vi "U3 - Create All Message Queues.vi"(8 "error in (no error)":errorcluster, 11 "Process Name":string="Feed Module 1") -> (0 "error out":errorcluster, 3 "Message Queues out":T1)   [LabVIEW 2018]
uses:
  support/Message Queue/Message Cluster.ctl
  support/Message Queue/Message Queue.lvlib
  support/Message Queue/All Message Queues.ctl
  support/Message Queue/Enqueue Message (Single).vi
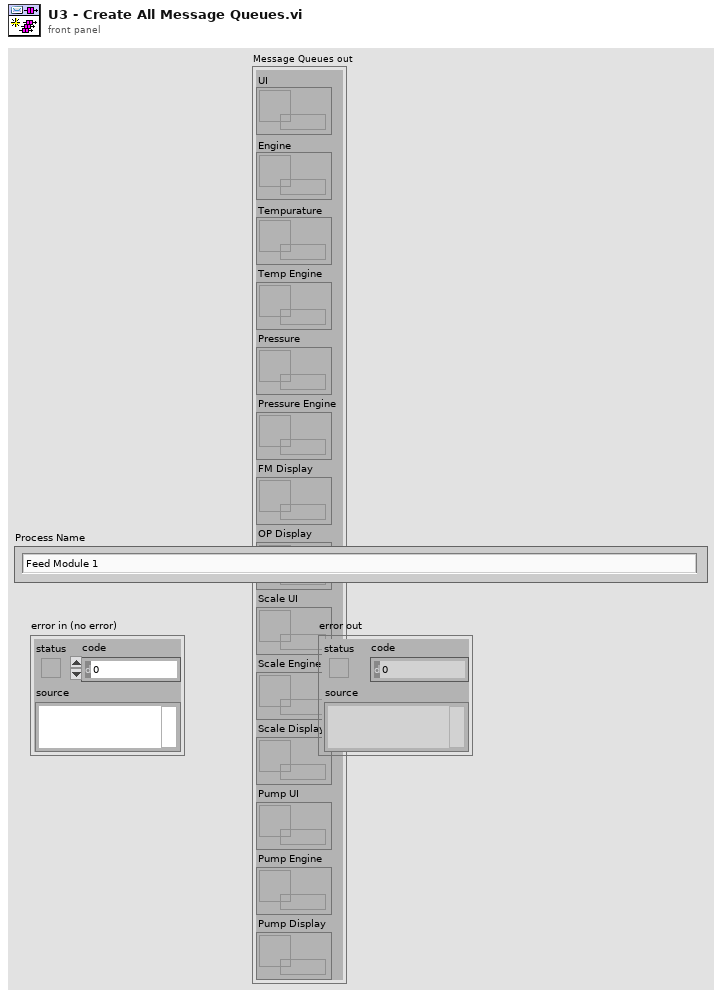
[diagram p1: front panel]
types:
  T1 = typedef "Message Queue.lvlib/All Message Queues.ctl" = cluster{"UI":refnum<queue>, "Engine":refnum<queue>, "Tempurature":refnum<queue>, "Temp Engine":refnum<queue>, "Pressure":refnum<queue>, "Pressure Engine":refnum<queue>, "FM Display":refnum<queue>, "OP Display":refnum<queue>, "Scale UI":refnum<queue>, "Scale Engine":refnum<queue>, "Scale Display":refnum<queue>, "Pump UI":refnum<queue>, "Pump Engine":refnum<queue>, "Pump Display":refnum<queue>}
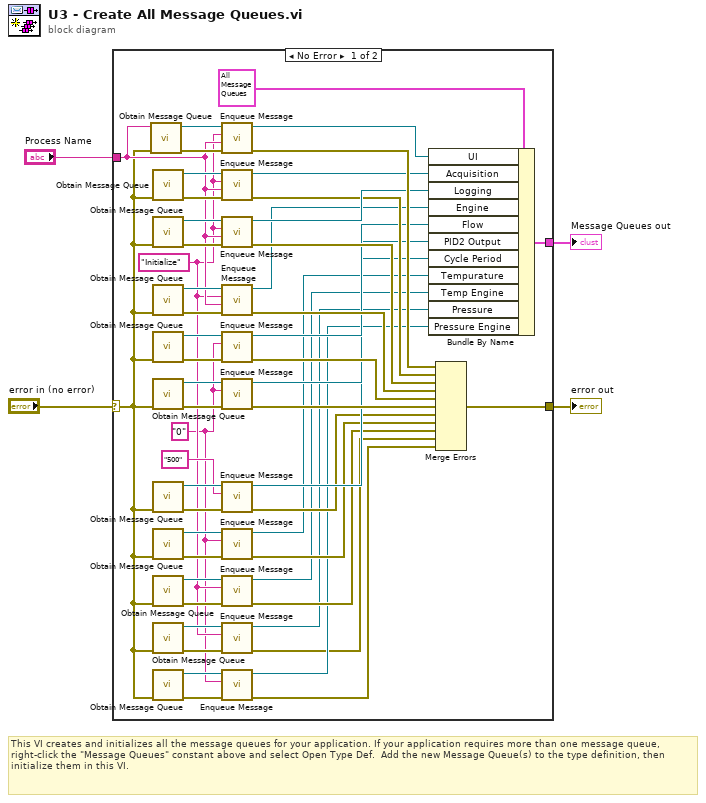
[diagram p0: block diagram]
diagram:
  # "This VI creates and initializes all the message queues for your application. If your application requires more than one message queue, right-click the \"Message Queues\" constant above and select Open Type Def.  Add the new Message Queue(s) to the type definition, then initialize them in this VI."
  n1 = case shown="No Error" "error in (no error)" {
    selector: "error in (no error)" -> [w9 w57]
    tunnel: [w44 w57] -> w4
    tunnel: [w54 _] -> w3
    tunnel: "Process Name" -> [w37 _]
    frame No Error {
      w5 = "0" ("Message")
      w6 = "Initialize" ("Message")
      n2 = call "Obtain Message Queue.vi"("error in (no error)"=w9, "name (unnamed)"=w37) -> ("error out"=w53:errorcluster, "Message Queue"=w52:refnum<queue>)  [unwired: 8 in]
      n3 = call "Obtain Message Queue.vi"("error in (no error)"=w9) -> ("error out"=w50:errorcluster, "Message Queue"=w51:refnum<queue>)  [unwired: 9 in]
      n4 = call "Obtain Message Queue.vi"("error in (no error)"=w9) -> ("error out"=w49:errorcluster, "Message Queue"=w48:refnum<queue>)  [unwired: 9 in]
      n5 = call "Obtain Message Queue.vi"("error in (no error)"=w9) -> ("error out"=w40:errorcluster, "Message Queue"=w41:refnum<queue>)  [unwired: 9 in]
      n6 = call "Obtain Message Queue.vi"("error in (no error)"=w9) -> ("error out"=w34:errorcluster, "Message Queue"=w36:refnum<queue>)  [unwired: 9 in]
      n7 = call "Obtain Message Queue.vi"("error in (no error)"=w9) -> ("error out"=w33:errorcluster, "Message Queue"=w35:refnum<queue>)  [unwired: 9 in]
      n8 = call "Obtain Message Queue.vi"("error in (no error)"=w9) -> ("error out"=w27:errorcluster, "Message Queue"=w28:refnum<queue>)  [unwired: 9 in]
      n9 = call "Obtain Message Queue.vi"("error in (no error)"=w9) -> ("error out"=w22:errorcluster, "Message Queue"=w23:refnum<queue>)  [unwired: 9 in]
      n10 = call "Obtain Message Queue.vi"("error in (no error)"=w9) -> ("error out"=w19:errorcluster, "Message Queue"=w18:refnum<queue>)  [unwired: 9 in]
      n11 = call "Obtain Message Queue.vi"("error in (no error)"=w9) -> ("error out"=w11:errorcluster, "Message Queue"=w10:refnum<queue>)  [unwired: 9 in]
      n12 = call "Obtain Message Queue.vi"("error in (no error)"=w9) -> ("error out"=w14:errorcluster, "Message Queue"=w15:refnum<queue>)  [unwired: 9 in]
      n13 = call-poly "Enqueue Message.vi"("error in (no error)"=w53, "Message Data"=w37, "Message"=w6, "Message Queue"=w52) -> ("error out"=w56:errorcluster, "dup Message Queue"=w47:refnum<queue>)  [unwired: 6 in]
      n14 = call-poly "Enqueue Message.vi"("error in (no error)"=w50, "Message Data"=w37, "Message"=w6, "Message Queue"=w51) -> ("error out"=w43:errorcluster, "dup Message Queue"=w46:refnum<queue>)  [unwired: 6 in]
      n15 = call-poly "Enqueue Message.vi"("error in (no error)"=w49, "Message Data"=w37, "Message"=w6, "Message Queue"=w48) -> ("error out"=w42:errorcluster, "dup Message Queue"=w45:refnum<queue>)  [unwired: 6 in]
      n16 = call-poly "Enqueue Message.vi"("error in (no error)"=w40, "Message Data"=w37, "Message"=w6, "Message Queue"=w41) -> ("error out"=w38:errorcluster, "dup Message Queue"=w39:refnum<queue>)  [unwired: 6 in]
      n17 = call-poly "Enqueue Message.vi"("error in (no error)"=w34, "Message"=w5, "Message Queue"=w36) -> ("error out"=w32:errorcluster, "dup Message Queue"=w30:refnum<queue>)  [unwired: 7 in]
      n18 = call-poly "Enqueue Message.vi"("error in (no error)"=w33, "Message"=w5, "Message Queue"=w35) -> ("error out"=w31:errorcluster, "dup Message Queue"=w29:refnum<queue>)  [unwired: 7 in]
      n19 = call-poly "Enqueue Message.vi"("error in (no error)"=w27, "Message"="500", "Message Queue"=w28) -> ("error out"=w24:errorcluster, "dup Message Queue"=w25:refnum<queue>)  [unwired: 7 in]
      n20 = call-poly "Enqueue Message.vi"("error in (no error)"=w22, "Message"=w5, "Message Queue"=w23) -> ("error out"=w20:errorcluster, "dup Message Queue"=w21:refnum<queue>)  [unwired: 7 in]
      n21 = call-poly "Enqueue Message.vi"("error in (no error)"=w19, "Message"=w6, "Message Queue"=w18) -> ("error out"=w16:errorcluster, "dup Message Queue"=w17:refnum<queue>)  [unwired: 7 in]
      n22 = call-poly "Enqueue Message.vi"("error in (no error)"=w11, "Message"=w6, "Message Queue"=w10) -> ("error out"=w7:errorcluster, "dup Message Queue"=w8:refnum<queue>)  [unwired: 7 in]
      n23 = call-poly "Enqueue Message.vi"("error in (no error)"=w14, "Message"=w5, "Message Queue"=w15) -> ("error out"=w12:errorcluster, "dup Message Queue"=w13:refnum<queue>)  [unwired: 7 in]
      n24 = Bundle By Name(cluster=T1 {"UI"=refnum, "Engine"=refnum, "Tempurature"=refnum, "Temp Engine"=refnum, "Pressure"=refnum, "Pressure Engine"=refnum, "FM Display"=refnum, "OP Display"=refnum, "Scale UI"=refnum, "Scale Engine"=refnum, "Scale Display"=refnum, "Pump UI"=refnum, "Pump Engine"=refnum, "Pump Display"=refnum} ("Message Queues"), "UI"=w47, "Acquisition"=w46, "Logging"=w45, "Engine"=w39, "Flow"=w30, "PID2 Output"=w29, "Cycle Period"=w25, "Tempurature"=w21, "Temp Engine"=w17, "Pressure"=w8, "Pressure Engine"=w13) -> (w54:T1)
      n25 = Merge Errors(w56, w43, w42, w38, w32, w31, w24, w20, w16, w7, w12) -> (w44:errorcluster)
    }
    frame Error {
    }
  }
  "Message Queues out" <- w3
  "error out" <- w4
